vi "FlatToRichmeasurement_DataRequest.vi"(5 "OutputClusterType":T1, 11 "InputCluster":T2) -> (3 "OutputCluster":T1)   [LabVIEW 2021, in "Measurement_server.lvlib"]
uses:
  Measurement_server.lvlib
  measurement_DataRequest_Flat.ctl
  measurement_DataRequest.ctl
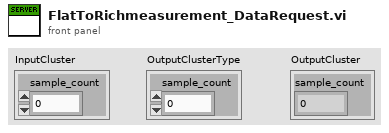
[diagram p1: front panel]
types:
  T1 = typedef "Measurement_server.lvlib/measurement_DataRequest.ctl" = cluster{"sample_count":i32}
  T2 = typedef "Measurement_server.lvlib/measurement_DataRequest_Flat.ctl" = cluster{"sample_count":i32}
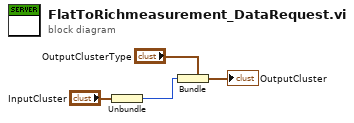
[diagram p0: block diagram]
diagram:
  n1 = Unbundle "Unbundle"("InputCluster") -> ("sample_count"=w1:i32)
  n2 = Bundle "Bundle"(cluster="OutputClusterType", "sample_count"=w1) -> (→"OutputCluster":T1)
